vi "Phasor Add Ticks to SEPL.vi"(1 "Ticks Calibrated s's":ext[](array[numeric]), 2 "Ticks Calibrated g's":ext[](array[numeric]), 3 "Ticks Lifetimes":ext[](array[numeric]), 5 "Lifetime Array in":ext[](array[numeric]), 7 "Calibrated g Array in":ext[](array[numeric]), 9 "Calibrated s Array in":ext[](array[numeric]), 11 "error in (no error)":errorcluster, 12 "Tick Length":dbl=0.01) -> (6 "Lifetime Array out":ext[](array[numeric]), 8 "Calibrated g Array out":ext[](array[numeric]), 10 "Calibrated s Array out":ext[](array[numeric]), 14 "Tick Labels (g,s))":T1[](array[typedef]), 15 "error out":errorcluster)   [LabVIEW 2021, in "Phasor.lvlib"]
uses:
  Phasor SEPL Tick Data.ctl
  Phasor (g, s).ctl
  Phasor.lvlib
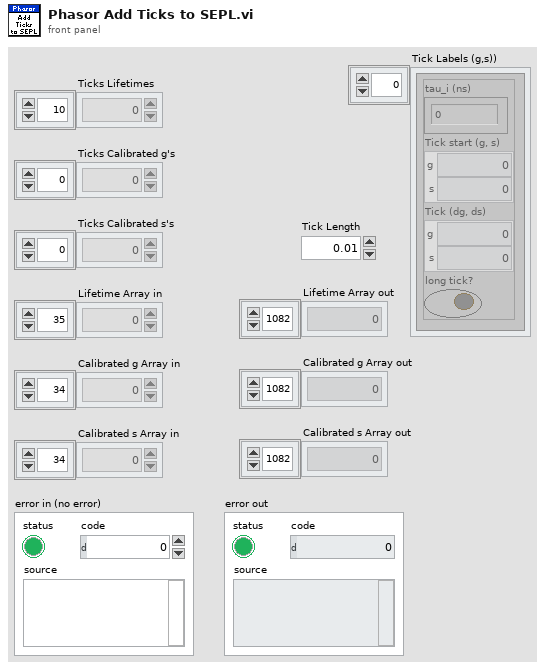
[diagram p1: front panel]
types:
  T1 = typedef "Phasor.lvlib/Phasor SEPL Tick Data.ctl" = cluster{"tau_i (ns)":dbl, "Tick start (g, s)":T2, "Tick (dg, ds)":T2, "long tick?":bool}
  T2 = typedef "Phasor.lvlib/Phasor (g, s).ctl" = cluster{"g":dbl, "s":dbl}
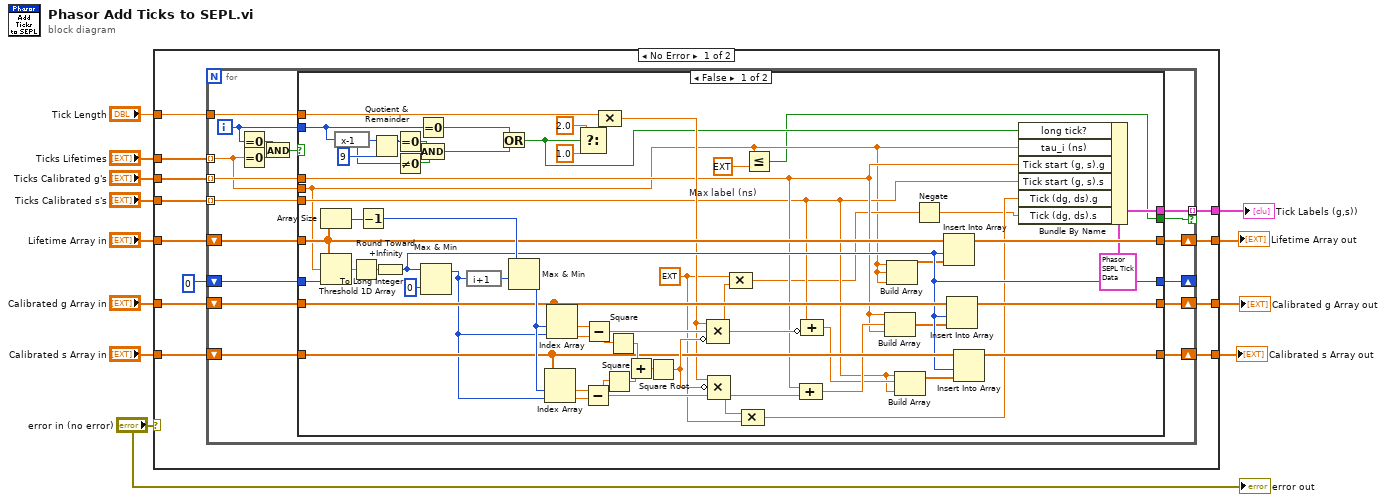
[diagram p0: block diagram]
diagram:
  n1 = case shown="No Error" "error in (no error)" {
    tunnel: "Ticks Lifetimes" -> [w24 _]
    tunnel: "Ticks Calibrated g's" -> [w23 _]
    tunnel: "Ticks Calibrated s's" -> [w22 _]
    tunnel: "Lifetime Array in" -> [w21 w107]
    tunnel: "Calibrated g Array in" -> [w20 w106]
    tunnel: "Calibrated s Array in" -> [w19 w105]
    tunnel: [w18 w107] -> w6
    tunnel: [w17 w106] -> w5
    tunnel: [w16 w105] -> w4
    tunnel: "Tick Length" -> [w14 _]
    tunnel: [w13 _] -> w1
    frame No Error {
      n2 = for {
        tunnel: w24 -> [w31] mode=indexing
        tunnel: w23 -> [w32] mode=indexing
        tunnel: w22 -> [w33] mode=indexing
        shift-right: [w37] -> w18
        shift-left: w21 -> [w38]
        shift-right: [w39] -> w17
        shift-left: w20 -> [w40]
        shift-right: [w35] -> w16
        shift-left: w19 -> [w36]
        shift-right: [w34] -> _
        shift-left: 0 -> [w42]
        tunnel: w14 -> [w41]
        tunnel: [w25] -> w13 mode=indexing if=w26
        i -> [w30]
        n3 = Equal To 0?(x=w30) -> (x = 0?=w29:bool)
        n4 = Equal To 0?(x=w31) -> (x = 0?=w28:bool)
        n5 = And(x=w29, y=w28) -> (x .and. y?=w27:bool)
        n6 = case shown="False" w27 {
          tunnel: w42 -> [w100 w103]
          tunnel: w41 -> [w81 _]
          tunnel: w40 -> [w74 w102]
          tunnel: [w73 w102] -> w39
          tunnel: w38 -> [w72 w104]
          tunnel: [w71 w104] -> w37
          tunnel: w36 -> [w70 w101]
          tunnel: [w69 w101] -> w35
          tunnel: [w68 w103] -> w34
          tunnel: w31 -> [w45 _]
          tunnel: w33 -> [w50 _]
          tunnel: w32 -> [w51 _]
          tunnel: w30 -> [w82 _]
          tunnel: [w43 _] -> w26
          tunnel: [w53 _] -> w25
          frame False {
            w44 = ext 10.0  # Max label (ns)
            w46 = ext 1.20000000000000000004 ("value")
            n7 = Array Size(array=w72) -> (size(s)=w98:i32)
            n8 = Threshold 1D Array(1:w100, 2:w45, 3:w72) -> (0:w60:ext)
            n9 = expression code="x-1"(w82) -> (w88:i32)
            n10 = Round Toward +Infinity(x=w60) -> (ceil(x): smallest int >= x=w59:ext)
            n11 = Decrement(x=w98) -> (x-1=w97:i32)
            n12 = Quotient & Remainder(x=w88, y=9 ("# Decades")) -> (x-y*floor(x/y)=w83:i32)  [unwired: 1 out]
            n13 = To Long Integer(number=w59) -> (32bit integer=w68:i32)
            n14 = Equal To 0?(x=w83) -> (x = 0?=w87:bool)
            n15 = Not Equal To 0?(x=w88) -> (x != 0?=w90:bool)
            n16 = Equal To 0?(x=w82) -> (x = 0?=w62:bool)
            n17 = Max & Min(x=w68, y=0) -> (max(x,y)=w63:i32)  [unwired: 1 out]
            n18 = Compound Arithmetic op=AND(w87, w90) -> (w89:bool)
            n19 = expression code="i+1"(w63) -> (w61:i32)
            n20 = Or(x=w62, y=w89) -> (x .or. y?=w52:bool)
            n21 = Max & Min(x=w97, y=w61) -> (min(x,y)=w96:i32)  [unwired: 1 out]
            n22 = Index Array(array=w70, index #1=w96, index #2=w63) -> (element #1=w93:ext, element #2=w92:ext)
            n23 = Index Array(array=w74, index #1=w96, index #2=w63) -> (element #1=w95:ext, element #2=w94:ext)
            n24 = Select(t=2.0 ("value"), s=w52, f=1.0) -> (s? t:f=w86:dbl)
            n25 = Subtract(x=w93, y=w92) -> (x-y=w76:ext)
            n26 = Subtract(x=w95, y=w94) -> (x-y=w77:ext)
            n27 = Compound Arithmetic op=MULTIPLY(w81, w86) -> (w67:dbl)
            n28 = Square(x=w76) -> (x^2=w80:ext)
            n29 = Square(x=w77) -> (x^2=w79:ext)
            n30 = Add(x=w79, y=w80) -> (x+y=w78:ext)
            n31 = Square Root(x=w78) -> (sqrt(x)=w75:ext)
            n32 = Compound Arithmetic op=MULTIPLY(w67, w77, invert w75) -> (w56:ext)
            n33 = Compound Arithmetic op=MULTIPLY(w67, invert w75, w76) -> (w55:ext)
            n34 = Compound Arithmetic op=MULTIPLY(w46, w56) -> (w48:ext)
            n35 = Compound Arithmetic op=MULTIPLY(w55, w46) -> (w49:ext)
            n36 = Less Or Equal?(x=w45, y=w44) -> (x <= y?=w43:bool)
            n37 = Compound Arithmetic op=ADD(w51, w55) -> (w58:ext)
            n38 = Compound Arithmetic op=ADD(w50, invert w56) -> (w57:ext)
            n39 = Build Array(w51, w58, w51) -> (w65:ext[])
            n40 = Build Array(w45, w45, w45) -> (w66:ext[])
            n41 = Build Array(w50, w57, w50) -> (w64:ext[])
            n42 = Negate(x=w48) -> (-x=w47:ext)
            n43 = Insert Into Array(array=w72, index=w68, new element=w66) -> (w71:ext[])
            n44 = Insert Into Array(array=w74, index=w68, new element=w65) -> (w73:ext[])
            n45 = Insert Into Array(array=w70, index=w68, new element=w64) -> (w69:ext[])
            n46 = Bundle By Name(cluster=T1 {"tau_i (ns)"=0.0, "Tick start (g, s)"={"g"=0.0, "s"=0.0}, "Tick (dg, ds)"={"g"=0.0, "s"=0.0}, "long tick?"=FALSE}, "long tick?"=w52, "tau_i (ns)"=w45, "Tick start (g, s).g"=w51, "Tick start (g, s).s"=w50, "Tick (dg, ds).g"=w49, "Tick (dg, ds).s"=w47) -> (w53:T1)
          }
          frame True {
            # "skip first tick if tau = 0, as it is sometimes problematic"
          }
        }
      }
    }
    frame Error {
    }
  }
  "Calibrated s Array out" <- w4
  "Calibrated g Array out" <- w5
  "Lifetime Array out" <- w6
  "Tick Labels (g,s))" <- w1
  "error out" <- "error in (no error)"
